vi "Snake_Eyes.vi"() -> ()   [LabVIEW 2022 SP3]
uses:
  <vilib>/numeric/Random Number (Range) I64.vi
  <vilib>/numeric/sub_Random U32.vi
panel:
  out "Number of Rolls":i32
  out "Same Value?":bool=TRUE
  out "Dice #2":i32
  out "Dice #1":i32
  # "Snake_Eyes:\nThis program simulates the rolling of 2 dice.\nIf the values are equal, the green light will\nlight. If they are not equal, they will roll again."
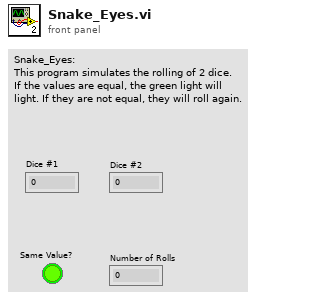
[diagram p1: front panel]
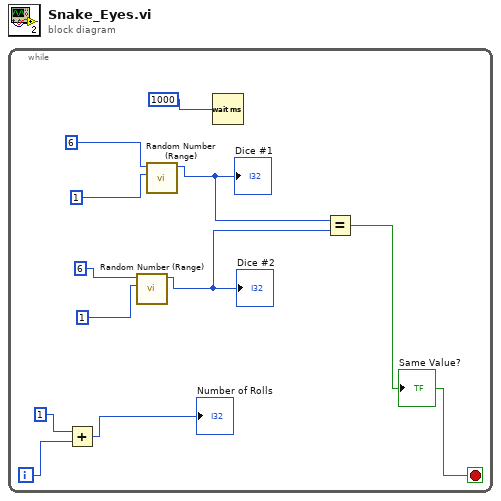
[diagram p0: block diagram]
diagram:
  n1 = while {
    i -> [w3]
    stop <- w5 stop-if-true
    n2 = Add(x=1, y=w3) -> (x+y=→"Number of Rolls":i32)
    n3 = call-poly <vilib>:"Random Number (Range).vi"("lower bound (-100)"=1, "upper bound (100)"=6) -> ("number"=w6:i64)  [unwired: 9 in]
    "Dice #2" <- w6
    n4 = call-poly <vilib>:"Random Number (Range).vi"("lower bound (-100)"=1, "upper bound (100)"=6) -> ("number"=w7:i64)  [unwired: 9 in]
    "Dice #1" <- w7
    n5 = Wait (ms)(milliseconds to wait=1000) -> ()  [unwired: 1 out]
    n6 = Equal?(x=w7, y=w6) -> (x = y?=w5:bool)
    "Same Value?" <- w5
  }
